vi "Update_Position_Test.vi"() -> ()   [LabVIEW 2016]
panel:
  out "Angle":dbl
  out "Robot Y Location":dbl
  out "Robot X Location":dbl
  in  "Run":bool
  in  "Motor On Duration":dbl
  in  "Motor 2 Value":dbl
  in  "Motor 1 Value":dbl
  in  "Robot Length":dbl
  in  "Robot Width":dbl
  in  "Robot Y Location":dbl
  in  "Robot X Location":dbl
  in  "Angle":dbl
  out "Robot Position":cluster{dbl[], dbl[]}[](graph)
  # "in"
  # "in"
  # "in"
  # "in"
  # "degrees"
  # "s"
  # "in"
  # "in"
  # "degrees"
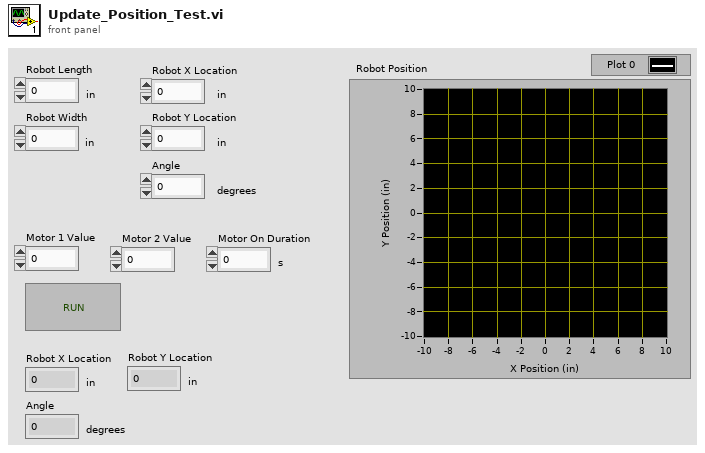
[diagram p1: front panel]
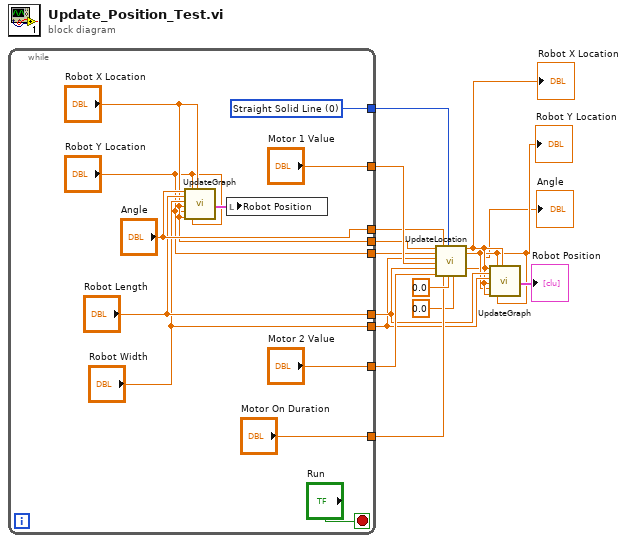
[diagram p0: block diagram]
diagram:
  n1 = while {
    tunnel: [w26] -> w14
    tunnel: ["Motor 1 Value"] -> w13
    tunnel: ["Motor 2 Value"] -> w12
    tunnel: ["Motor On Duration"] -> w10
    tunnel: ["Angle"] -> w9
    tunnel: ["Robot Length"] -> w8
    tunnel: ["Robot Width"] -> w7
    tunnel: ["Robot X Location"] -> w6
    tunnel: ["Robot Y Location"] -> w5
    stop <- "Run" stop-if-true
    w26 = u16 0 items=["Straight Solid Line", "Straigh Dotted Line", "Straight Broken Line", "Curved Solid Line", "Curved Dotted Line", "Curved Broken Line"] ("Select Track")
    n2 = call "UpdateGraph.vi"("Angle"="Angle", "Robot Length"="Robot Length", "Robot Width"="Robot Width", "Sensor 1 X"="Robot X Location", "Sensor 1 Y"="Robot Y Location", "Sensor 2 X"="Robot X Location", "Robot Y"="Robot Y Location", "Sensor 2 Y"="Robot Y Location", "Robot X"="Robot X Location") -> ("appended array"=w22:cluster{dbl[], dbl[]}[])  [unwired: 10 in]
    n3 = local write "Robot Position"(w22) -> ()
  }
  n4 = call "UpdateLocation.vi"("Robot X Location"=w6, "Robot Y Location"=w5, "Robot Width"=w7, "Motor 1 Value"=w13, "Robot Length"=w8, "Motor 2 Value"=w12, "Angle"=w9, "Motor On Duration"=w10, "Select Track"=w14, "Motor 1 Error"=0.0, "Motor 2 Error"=0.0 ("Motor 1 Error")) -> ("New Robot X Location"=w4:dbl, "New Robot Y Location"=w3:dbl, "New Angle"=w2:dbl)  [unwired: 4 in, 2 out]
  "Robot X Location" <- w4
  "Angle" <- w2
  "Robot Y Location" <- w3
  n5 = call "UpdateGraph.vi"("Angle"=w2, "Robot Length"=w8, "Robot Width"=w7, "Sensor 1 X"=w4, "Sensor 1 Y"=w3, "Sensor 2 X"=w4, "Robot Y"=w3, "Sensor 2 Y"=w3, "Robot X"=w4) -> ("appended array"=→"Robot Position":cluster{dbl[], dbl[]}[])  [unwired: 10 in]
